vi "SendVoltage.vi"(1 "value":sgl format="%0.2f", 2 "error in (no error)":errorcluster, 3 "DAQmx Global Channel":refnum<k21>="Voltage top piezo laser") -> (0 "error out":errorcluster)   [LabVIEW 2017]
uses:
  <vilib>/DAQmx/write.llb/DAQmx Write (Analog DBL 1Chan 1Samp).vi
  <vilib>/DAQmx/miscellaneous.llb/DAQmx Fill In Error Info.vi
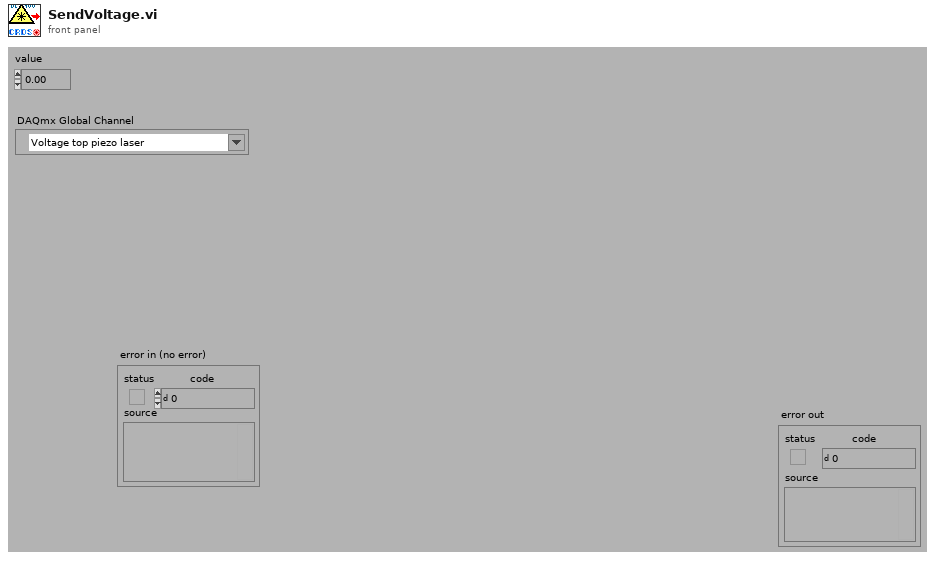
[diagram p1: front panel]
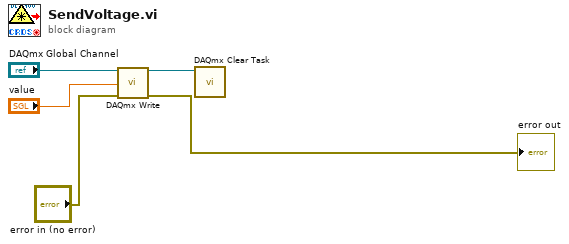
[diagram p0: block diagram]
diagram:
  n1 = call-poly <vilib>:"DAQmx Write.vi"("task/channels in"="DAQmx Global Channel", "data"="value", "error in"="error in (no error)") -> ("task out"=w3:refnum<k21>, "error out"=→"error out":errorcluster)  [unwired: 1 in, 10 out]
  n2 = call <vilib>:"DAQmx Clear Task.vi"("task in"=w3) -> ()  [unwired: 1 in, 14 out]
